vi "UpdateDropletTable.vi"(8 "error in (no error)":errorcluster) -> (0 "error out":errorcluster, 3 "DropletTabeVariant":variant)   [LabVIEW 2013]
doc: "Use this template to build a VI to use as a subVI."
uses:
  DB/DbEnum.ctl
  DB/DropletDB.ctl
  TypeDef/DropletDisplay.ctl
  <vilib>/vision/Image Controls.llb/IMAQ Image.ctl
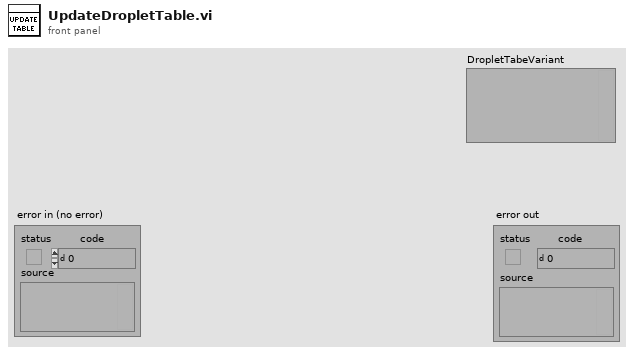
[diagram p1: front panel]
types:
  T1 = typedef "DropletDB.ctl" = cluster{"ImageFreezeIndex":i32, "DropIndex":i32, "Position":cluster{"x":sgl, "y":sgl}, "Bounding Box":cluster{"x":sgl, "y":sgl}[], "Score":sgl, "GreyLevelInBoundingBox":dbl[], "GLDifference":dbl[], "Baseline level":dbl, "Peak":cluster{"Value":dbl, "Index":u32}, "Peak Onset":cluster{"Value":dbl, "Index":u32}, "FreezeFileName":string, "FreezeAbsTime":timestamp, "FreezeRelTime(sec)":u32, "FreezeTemperature":dbl, "ImageIndexArray":u32[], "Freeze Point Found":bool, "Baseline std":dbl, "FreezedImageArray":cluster{"Image":u8[][]}[]}[]
  T2 = typedef "DbEnum.ctl" = enum16{"Init", "Insert Detection Result Data", "Insert Grey Level Result", "Insert Baseline Results", "AddFreezeImagesAtCertainDroplet", "Insert Freeze Analysis Results", "GetDropDB", "GetNoFreezedDroplets", "GetGreyLevelAndDiff", "GetGreyLevelatIndexTime", "GetDropletsBoundingBox"}
  T3 = typedef "DropletDisplay.ctl" = cluster{"Drop Info":dbl[], "Freeze Images":T4[], "Include Droplet":bool, "Remark":string}[]
  T4 = typedef "IMAQ Image.ctl" = refnum<image>
  T5 = cluster{"Drop Info":dbl[], "Freeze Images":T4[], "Include Droplet":bool, "Remark":string}
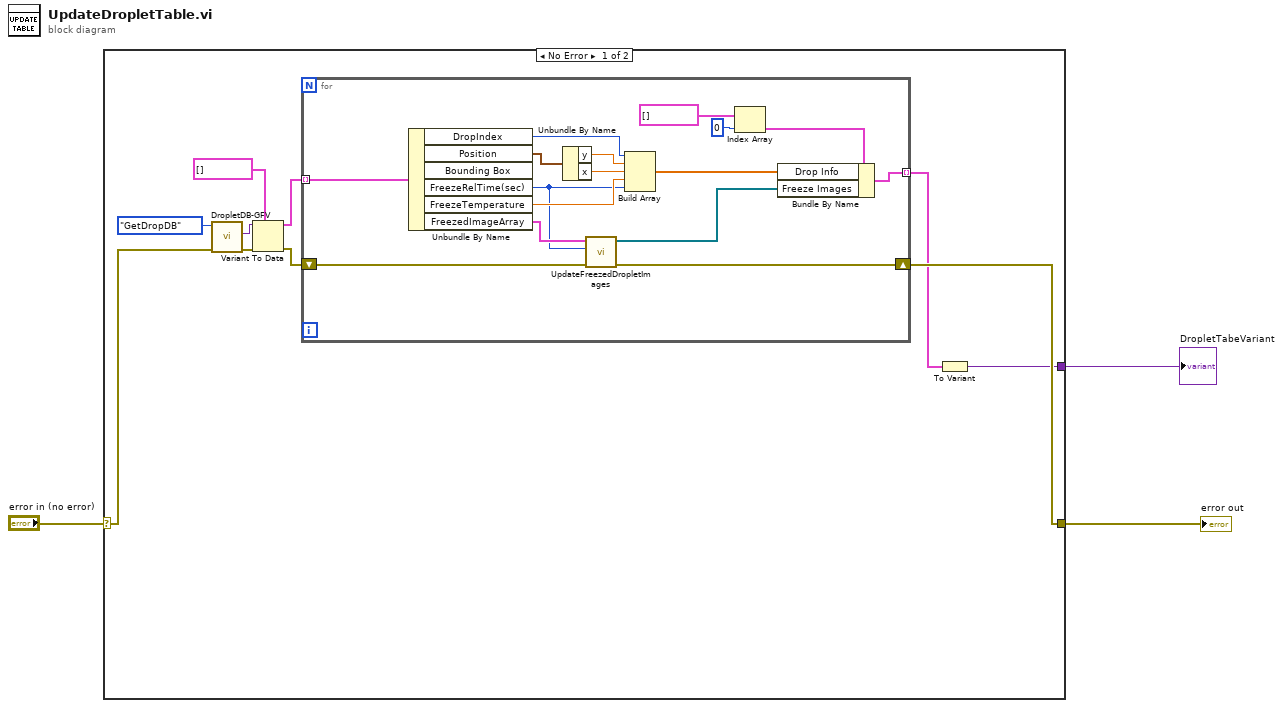
[diagram p0: block diagram]
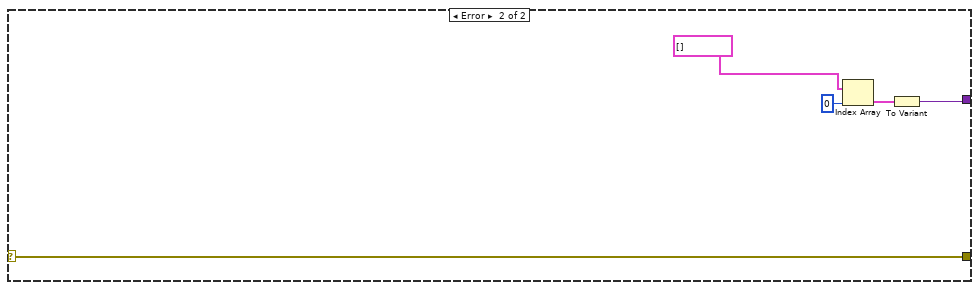
[diagram p2: hidden frame]
diagram:
  n1 = case shown="No Error" "error in (no error)" {
    selector: "error in (no error)" -> [w5 w34]
    tunnel: [w8 w34] -> w2
    tunnel: [w6 w31] -> w1
    frame No Error {
      n2 = call "DropletDB-GFV.vi"("error in (no error)"=w5, "Command In"=DbEnum."GetDropDB") -> ("error out"=w12:errorcluster, "Data out"=w13:variant)  [unwired: 8 in]
      n3 = Variant To Data(error in=w12, type=T1 [] ("DropletArray"), Variant=w13) -> (data=w10:T1, error out=w4:errorcluster)
      n4 = for {
        tunnel: w10 -> [w29] mode=indexing
        shift-right: [w17] -> w8
        shift-left: w4 -> [w18]
        tunnel: [w25] -> w7 mode=indexing
        n5 = Unbundle By Name(w29) -> ("DropIndex"=w19:i32, "Position"=w24:cluster{"x":sgl, "y":sgl}, "FreezeRelTime(sec)"=w15:u32, "FreezeTemperature"=w21:dbl, "FreezedImageArray"=w16:cluster{"Image":u8[][]}[])  [unwired: 1 out]
        n6 = Unbundle By Name(w24) -> ("y"=w23:sgl, "x"=w22:sgl)
        n7 = call "UpdateFreezedDropletImages.vi"("error in (no error)"=w18, "FreezeRelTime(sec)"=w15, "FreezedImageArray"=w16) -> ("error out"=w17:errorcluster, "OutputFreezedImagesRef"=w14:T4[])  [unwired: 7 in]
        n8 = Build Array(w19, w23, w22, w21, w15) -> (w20:dbl[])
        n9 = Index Array(array=T3 [] ("Droplet Display"), index=0) -> (element=w26:T5)
        n10 = Bundle By Name(cluster=w26, "Drop Info"=w20, "Freeze Images"=w14) -> (w25:T5)
      }
      n11 = To Variant(anything=w7) -> (Variant=w6:variant)
    }
    frame Error {
      n12 = Index Array(array=T3 [] ("Droplet Display"), index=0) -> (element=w30:T5)
      n13 = To Variant(anything=w30) -> (Variant=w31:variant)
    }
  }
  "error out" <- w2
  "DropletTabeVariant" <- w1
